vi "CRYDistance between two points.vi"(10 "Point B":cluster{"X":dbl, "Y":dbl} {"Y" format="%.2f"; "X" format="%.2f"}, 11 "Point A":cluster{"X":dbl, "Y":dbl} {"Y" format="%.2f"; "X" format="%.2f"}) -> (3 "Distance A to B":dbl format="%.2f")   [LabVIEW 2013]
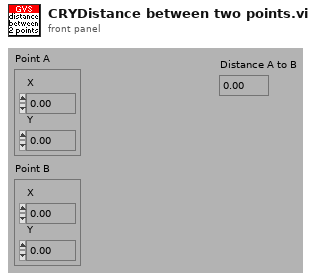
[diagram p1: front panel]
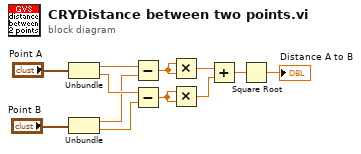
[diagram p0: block diagram]
diagram:
  n1 = Unbundle("Point A") -> ("X"=w7:dbl, "Y"=w9:dbl)
  n2 = Unbundle("Point B") -> ("X"=w8:dbl, "Y"=w10:dbl)
  n3 = Subtract(x=w7, y=w8) -> (x-y=w6:dbl)
  n4 = Subtract(x=w9, y=w10) -> (x-y=w5:dbl)
  n5 = Multiply(x=w6, y=w6) -> (x*y=w4:dbl)
  n6 = Multiply(x=w5, y=w5) -> (x*y=w3:dbl)
  n7 = Add(x=w4, y=w3) -> (x+y=w2:dbl)
  n8 = Square Root(x=w2) -> (sqrt(x)=→"Distance A to B":dbl)
